vi "BuildPlotColorsBands.vi"(5 "Labels":string[](array[string]), 6 "View Type":u16(ring) items=["As measured", "Normalize", "Separate", "Cplx Average", "Real Average", "Standard Deviation"], 7 "Colors":u32[](array[numeric]), 8 "error in (no error)":errorcluster, 9 "Bands":u16, 11 "WaveformGraph in":refnum<vi>) -> (3 "WaveformGraph out":refnum<vi>)   [LabVIEW 2022 SP3]
uses:
  Mic/Mic_Global.vi
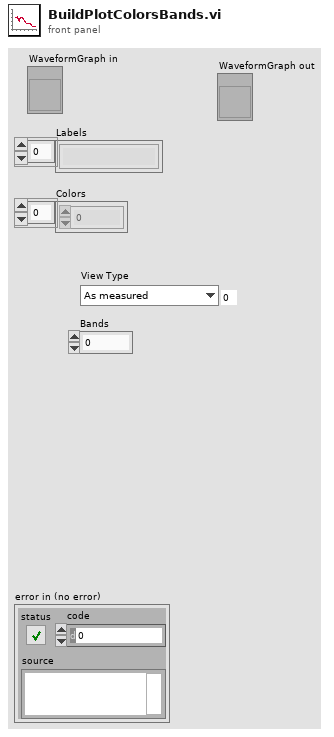
[diagram p1: front panel]
types:
  T1 = cluster{"Alerts":bool, "Log X Axis":bool, "dB scale":bool, "Averaging":bool, "Fade":dbl, "Centroids?":bool, "line thickness":u8}
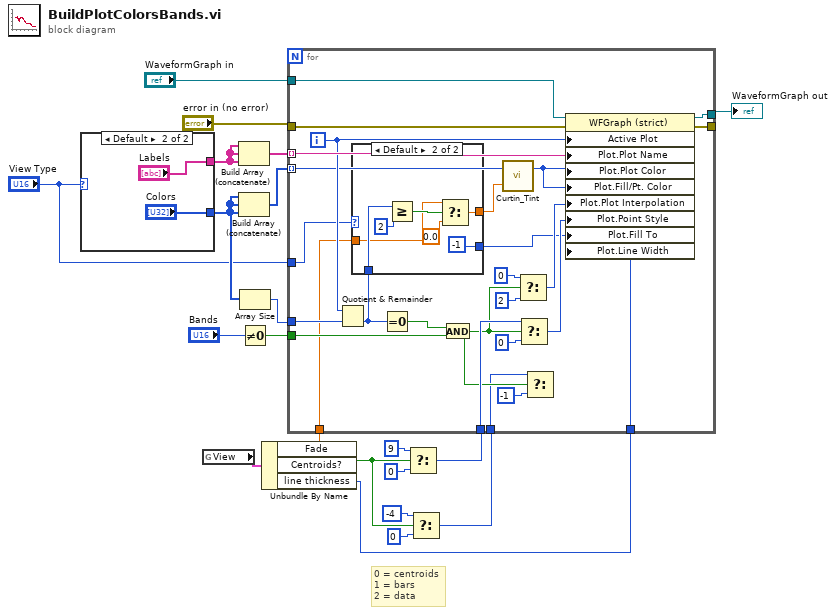
[diagram p0: block diagram]
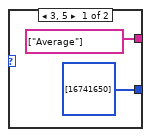
[diagram p2: hidden frame]
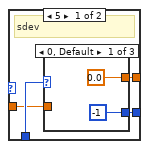
[diagram p3: hidden frame]
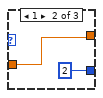
[diagram p4: hidden frame]
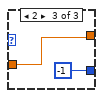
[diagram p5: hidden frame]
diagram:
  # "0 = centroids\n1 = bars\n2 = data"
  n1 = case shown="Default" "View Type" {
    tunnel: [string[] ["Average"] ("Labels") "Labels"] -> w13
    tunnel: [u32[] [16741650] ("Colors") "Colors"] -> w12
    frame 3, 5 {
    }
    frame Default {
    }
  }
  n2 = global read "Mic_Global.vi" "View"() -> (w11:T1)
  n3 = Build Array (concatenate)(w13, w13, w13) -> (w18:string[])
  n4 = Build Array (concatenate)(w12, w12, w12) -> (w15:u32[])
  n5 = Array Size(array=w12) -> (size(s)=w16:i32)
  n6 = Not Equal To 0?(x="Bands") -> (x != 0?=w21:bool)
  n7 = Unbundle By Name(w11) -> ("Fade"=w7:dbl, "Centroids?"=w4:bool, "line thickness"=w1:u8)
  n8 = Select(t=9 ("y"), s=w4, f=0 ("y")) -> (s? t:f=w8:i32)
  n9 = Select(t=-4 ("y"), s=w4, f=0 ("y")) -> (s? t:f=w3:i32)
  n10 = for {
    tunnel: w15 -> [w35] mode=indexing
    tunnel: "WaveformGraph in" -> [w51]
    tunnel: w16 -> [w44]
    tunnel: "error in (no error)" -> [w49]
    tunnel: [w48] -> _
    tunnel: w18 -> [w47] mode=indexing
    tunnel: [w46] -> w19
    tunnel: w21 -> [w43]
    tunnel: w8 -> [w34]
    tunnel: w7 -> [w33]
    tunnel: w3 -> [w30]
    tunnel: "View Type" -> [w29]
    tunnel: w1 -> [w26]
    i -> [w45]
    n11 = Quotient & Remainder(x=w45, y=w44) -> (floor(x/y)=w42:i32)  [unwired: 1 out]
    n12 = case shown="Default" w29 {
      tunnel: [w53 w68] -> w50
      tunnel: w42 -> [w54 w64]
      tunnel: w33 -> [w52 w63]
      tunnel: [w55 i16 -1 ("Plot.Fill To")] -> w28
      frame 5 {
        # "sdev"
        n13 = case shown="0, Default" w54 {
          tunnel: [i16 -1 ("Plot.Fill To") i16 2 ("Plot.Fill To") i16 -1 ("Plot.Fill To")] -> w55
          tunnel: [0.0 ("t") w58 w60] -> w53
          tunnel: w52 -> [_ w58 w60]
          frame 0, Default {
          }
          frame 1 {
          }
          frame 2 {
          }
        }
      }
      frame Default {
        n14 = Greater Or Equal?(x=w64, y=2) -> (x >= y?=w66:bool)
        n15 = Select(t=w63, s=w66, f=0.0 ("t")) -> (s? t:f=w68:dbl)
      }
    }
    n16 = Equal To 0?(x=w42) -> (x = 0?=w41:bool)
    n17 = And(x=w41, y=w43) -> (x .and. y?=w31:bool)
    n18 = call "Curtin_Tint.vi"("Tint Factor"=w50, "Plot.Plot Color"=w35) -> ("Plot.Plot Color 2"=w27:u32)  [unwired: 1 in]
    n19 = Select(t=0 ("y"), s=w31, f=2 ("y")) -> (s? t:f=w36:i32)
    n20 = Select(t=w34, s=w31, f=0 ("y")) -> (s? t:f=w39:i32)
    n21 = Select(t=w30, s=w31, f=-1 ("y")) -> ()  [unwired: 1 out]
    n22 = property on="Property Node" class="WFGraph (strict)"(reference=w51, error in=w49, "Active Plot"=w45, "Plot.Plot Name"=w47, "Plot.Plot Color"=w27, "Plot.Fill/Pt. Color"=w27, "Plot.Plot Interpolation"=w36, "Plot.Point Style"=w39, "Plot.Fill To"=w28, "Plot.Line Width"=w26) -> (reference out=w46:refnum<vi>, error out=w48:errorcluster)
  }
  "WaveformGraph out" <- w19
